vi "Close References.vi"(8 "error in":errorcluster, 10 "References":T1, 11 "J1939 Cluster":T7) -> (0 "error out":errorcluster)   [LabVIEW 2015, in "J1939 Addon Engine.lvlib"]
uses:
  J1939 Addon Engine.lvlib
  Types/Setup Information Cluster.ctl
  <vilib>/xnet/xnet.llb/XNET Frame CAN.ctl
  <vilib>/xnet/xnet.llb/XNET Frame Type CAN.ctl
  Shared/J1939 Utilities/Types/CAN Outgoing Message Cluster.ctl
  Types/TP List References.ctl
  Types/BAM Buffer Connections List_Ref.ctl
  Types/TP Buffer Connection Cluster.ctl
  Types/Connection Mode Generation Connection Ref.ctl
  Types/Connection Mode Generation Connection Cluster.ctl
  Types/BAM Generation Connections List_Ref.ctl
  Types/BAM Generation Connection Cluster.ctl
  Types/Address Table Reference.ctl
  Types/RQST Lookup Table Reference.ctl
  Shared/J1939 Utilities/J1939 Utilities.lvlib
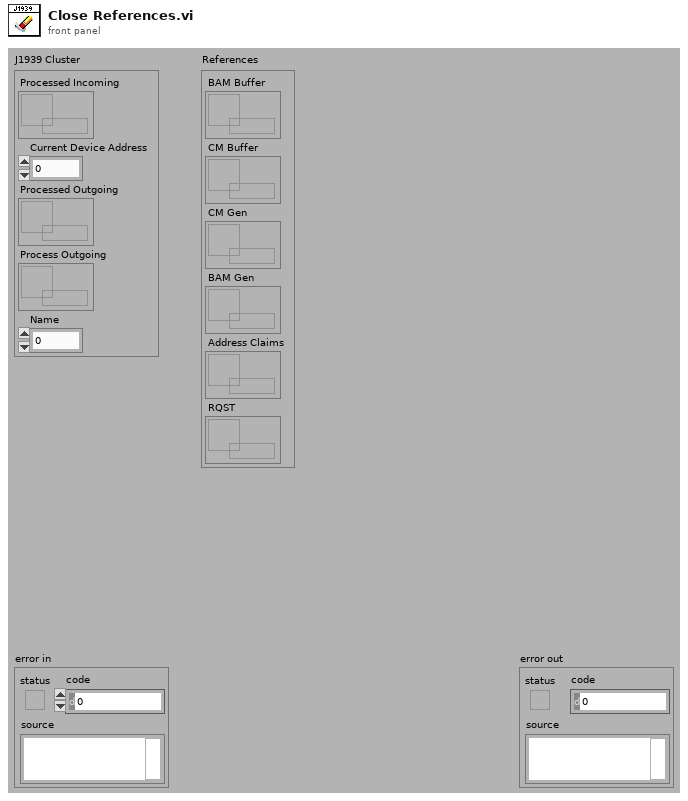
[diagram p1: front panel]
types:
  T1 = typedef "J1939 Addon Engine.lvlib/TP List References.ctl" = cluster{"BAM Buffer":T2, "CM Buffer":T2, "CM Gen":T3, "BAM Gen":T4, "Address Claims":T5, "RQST":T6}
  T2 = typedef "J1939 Addon Engine.lvlib/BAM Buffer Connections List_Ref.ctl" = refnum<data-value>
  T3 = typedef "J1939 Addon Engine.lvlib/Connection Mode Generation Connection Ref.ctl" = refnum<data-value>
  T4 = typedef "J1939 Addon Engine.lvlib/BAM Generation Connections List_Ref.ctl" = refnum<data-value>
  T5 = typedef "J1939 Addon Engine.lvlib/Address Table Reference.ctl" = refnum<data-value>
  T6 = typedef "J1939 Addon Engine.lvlib/RQST Lookup Table Reference.ctl" = refnum<data-value>
  T7 = typedef "J1939 Addon Engine.lvlib/Setup Information Cluster.ctl" = cluster{"Processed Incoming":refnum<queue>, "Current Device Address":u8, "Processed Outgoing":refnum<queue>, "Process Outgoing":refnum<queue>, "Name":u64}
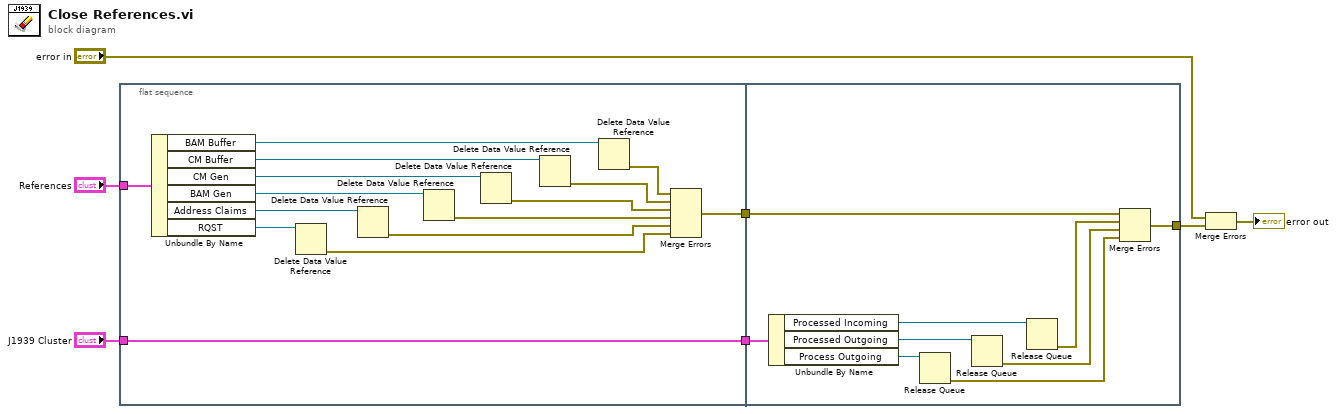
[diagram p0: block diagram]
diagram:
  n1 = flat-sequence {
    tunnel: "References" -> [w22]
    tunnel: [w15] -> w6
    tunnel: "J1939 Cluster" -> [w15]
    tunnel: [w8] -> w4
    tunnel: w6 -> [w31]
    tunnel: w4 -> [w27]
    tunnel: [w23] -> w3
    frame #0 {
      n2 = Unbundle By Name(w22) -> ("BAM Buffer"=w16:T2, "CM Buffer"=w17:T2, "CM Gen"=w18:T3, "BAM Gen"=w19:T4, "Address Claims"=w20:T5, "RQST"=w21:T6)
      n3 = Delete Data Value Reference(data value reference=w21) -> (error out=w9:errorcluster)  [unwired: 1 in, 1 out]
      n4 = Delete Data Value Reference(data value reference=w20) -> (error out=w10:errorcluster)  [unwired: 1 in, 1 out]
      n5 = Delete Data Value Reference(data value reference=w19) -> (error out=w11:errorcluster)  [unwired: 1 in, 1 out]
      n6 = Delete Data Value Reference(data value reference=w18) -> (error out=w12:errorcluster)  [unwired: 1 in, 1 out]
      n7 = Delete Data Value Reference(data value reference=w17) -> (error out=w13:errorcluster)  [unwired: 1 in, 1 out]
      n8 = Delete Data Value Reference(data value reference=w16) -> (error out=w14:errorcluster)  [unwired: 1 in, 1 out]
      n9 = Merge Errors(w14, w13, w12, w11, w10, w9) -> (w8:errorcluster)
    }
    frame #1 {
      n10 = Unbundle By Name(w31) -> ("Processed Incoming"=w28:refnum<queue>, "Processed Outgoing"=w29:refnum<queue>, "Process Outgoing"=w30:refnum<queue>)
      n11 = Release Queue(queue=w30) -> (error out=w24:errorcluster)  [unwired: 2 in, 2 out]
      n12 = Release Queue(queue=w29) -> (error out=w25:errorcluster)  [unwired: 2 in, 2 out]
      n13 = Release Queue(queue=w28) -> (error out=w26:errorcluster)  [unwired: 2 in, 2 out]
      n14 = Merge Errors(w27, w26, w25, w24) -> (w23:errorcluster)
    }
  }
  n15 = Merge Errors("error in", w3) -> (→"error out":errorcluster)
